vi "TLCCS Get Wavelength Data.vi"(8 "error in (no error)":errorcluster {"code" format="%.0x"}, 9 "Data Set (Factory Calibration Data)":i16(ring) items=["Factory Calibration Data", "User Calibration Data"], 11 "instrument handle":refnum<visa-resource-name>) -> (0 "error out":errorcluster {"code" format="%.0x"}, 1 "Minimum Wavelength (400)":dbl, 2 "Wavelength Data Array":dbl[](array[numeric]) format="%.2p", 3 "instrument handle out":refnum<visa-resource-name>, 4 "Maximum Wavelength (400)":dbl)   [LabVIEW 2020]
doc: "This VI returns data for the pixel-wavelength correlation.\nThe maximum and the minimum wavelength are additionally provided in two separate return values.\n\nNote:\nIf you do not need either of these values you may pass NULL.\n\n\nThe value returned in Wavelength_Data_Array[0] is the wavelength at pixel 1, this is also the minimum wavelength, the value returned in Wavelength_Data_Array[1] is the wavelength at pixel 2 and so on until Wavelength_Data_Array[CCS_SERIES_NUM_PIXELS-1] which provides the wavelength at pixel CCS_SERIES_NUM_PIXELS (3648). This is the maximum wavelength."
uses:
  tlccs_32.dll
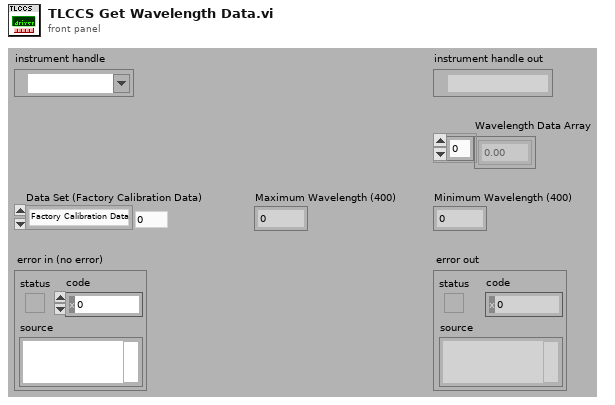
[diagram p1: front panel]
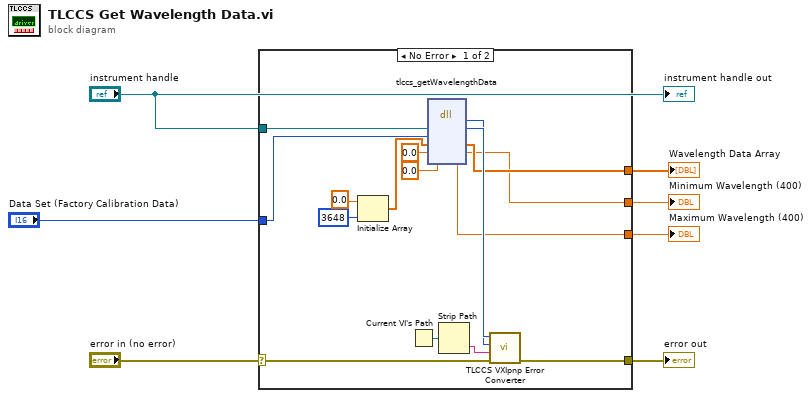
[diagram p0: block diagram]
diagram:
  n1 = case shown="No Error" "error in (no error)" {
    selector: "error in (no error)" -> [w18 w24]
    tunnel: [w17 w24] -> w7
    tunnel: "instrument handle" -> [w22 _]
    tunnel: "Data Set (Factory Calibration Data)" -> [w16 _]
    tunnel: [w12 _] -> w3
    tunnel: [w10 _] -> w2
    tunnel: [w8 _] -> w1
    frame No Error {
      n2 = Initialize Array(0.0 ("element"), 3648 ("dimension size")) -> (w15:dbl[])
      n3 = Current VI's Path() -> (path=w23:path)
      n4 = dll-call lib="tlccs_32.*" fn="tlccs_getWavelengthData"("Instrument Handle"=w22, "Data Set"=w16, "Wavelength Data Array"=w15, "Minimum Wavelength"=0.0, "Maximum Wavelength"=0.0) -> (w20:i32, "Instrument Handle"=w21:u32, "Wavelength Data Array"=w12:dbl[], "Minimum Wavelength"=w10:dbl, "Maximum Wavelength"=w8:dbl)  [unwired: 4 in, 2 out]
      n5 = Strip Path(path=w23) -> (name=w19:string)  [unwired: 1 out]
      n6 = call "TLCCS VXIpnp Error Converter.vi"("error in (no error)"=w18, "name of VI (\"\")"=w19, "CVI error code (0)"=w20, "instrument handle"=w21) -> ("error out"=w17:errorcluster)  [unwired: 6 in, 1 out]
    }
    frame Error {
    }
  }
  "error out" <- w7
  "Wavelength Data Array" <- w3
  "Minimum Wavelength (400)" <- w2
  "Maximum Wavelength (400)" <- w1
  "instrument handle out" <- "instrument handle"
